vi "CAN.Cleanup.vi"(8 "error in (no error)":errorcluster, 11 "State Variables Out":T1 {"ADCS Connection"."RX_DL" items=["8"=8, "12"=12, "16"=16, "20"=20, "24"=24, "32"=32, "48"=48, "64"=64]; "ADCS Connection"."TX_DL" items=["8"=8, "12"=12, "16"=16, "20"=20, "24"=24, "32"=32, "48"=48, "64"=64]; "ADCS Connection"."I/O Mode" items=["CAN", "CAN FD", "CAN FD+BRS"]; "Parameters"."Properties"."Writes"."Signals"."Byte Order" items=["Little Endian", "Big Endian"]; "Parameters"."Properties"."Writes"."Signals"."Data Type" items=["Signed", "Unsigned", "IEEE Float"]; "Parameters"."Properties"."CAN"."IO Mode" items=["CAN 2.0", "CAN FD", "CAN FD+BRS"]; "Parameters"."Properties"."CAN"."Fill Byte" format="%.0x"; "Parameters"."Properties"."CAN"."VW TP Channel ID" format="%.0x"; "Parameters"."Properties"."CAN"."Receive UUDT ID" format="%.0x"; "Parameters"."Properties"."CAN"."Receive Extension" format="%.0x"; "Parameters"."Properties"."CAN"."Transmit Extension" format="%.0x"; "Parameters"."Properties"."CAN"."Receive ID" format="%.0x"; "Parameters"."Properties"."CAN"."Transmit ID" format="%.0x"; "Parameters"."Properties"."Reads"."Signals"."Byte Order" items=["Little Endian", "Big Endian"]; "Parameters"."Properties"."Reads"."Signals"."Data Type" items=["Signed", "Unsigned", "IEEE Float"]}) -> (0 "error out":errorcluster)   [LabVIEW 2015, in "Diagnostics Addon Engine.lvlib"]
uses:
  Diagnostics Addon Engine.lvlib
  Types/Diagnostics.State.ctl
  <vilib>/NI/NIVS Addon Network Comm/Engine/VeriStand Comm.lvclass
  <vilib>/NI/NIVS Inline Async API/_VS Inline Async API/Process/Process.lvclass
  Shared/Types/SysDef.Compile.ctl
  Shared/Types/SysDef.Compile.Properties.ctl
  Shared/Types/CAN.ctl
  Shared/Types/CAN.Interface.ctl
  Shared/Types/Protocol.ctl
  Shared/Types/Transport.ctl
  Shared/Types/Security.ctl
  Shared/Types/986x.ctl
  Shared/Types/Frame.Compile.ctl
  Shared/Types/Type.ctl
  Shared/Types/Signal.ctl
  Shared/Types/DPID.ctl
  Shared/Types/DPID.Rate.ctl
  Shared/Types/DTC.Settings.ctl
  Shared/Types/DTC.Descriptor.ctl
  <vilib>/Automotive Diagnostic Command Set/Diagnostic Transport.llb/Diag Reference.ctl
  <vilib>/Automotive Diagnostic Command Set/Diagnostic Transport.llb/Transport Protocol Selector.ctl
  Types/XNET.Refs.ctl
  <vilib>/NI/AMC/Message Queue.ctl
  <vilib>/NI/AMC/Message.ctl
  <vilib>/NI/Tools/Keyed Array/KeyedArray.ctl
  <vilib>/NI/NIVS Inline Async API/_Data Access Engine/Data Access Engine/Types/Write.DVR.ctl
  <vilib>/NI/NIVS Inline Async API/_Data Access Engine/Access Type Classes/Write/Write.lvclass
  <vilib>/NI/NIVS Inline Async API/_Data Access Engine/Data Access Engine/Types/Read.DVR.ctl
  <vilib>/NI/NIVS Inline Async API/_Data Access Engine/Access Type Classes/Read/Read.lvclass
  <vilib>/NI/NIVS Inline Async API/_Data Access Engine/Data Access Engine/Types/ReadWrite.DVR.ctl
  <vilib>/NI/NIVS Inline Async API/_Data Access Engine/Access Type Classes/ReadWrite/ReadWrite.lvclass
  <vilib>/NI/NIVS Inline Async API/_Data Access Engine/Access Type Classes/Write/Write.lvclass/Write.ctl
  <vilib>/NI/NIVS Inline Async API/_Data Access Engine/Data Access Engine/Methods/Write.Data.vi
  <vilib>/NI/NIVS Inline Async API/_Data Access Engine/Access Type Classes/Write/Write.ProcessData.vi
  ADCS.Get.ErrorByte.vi
  <vilib>/xnet/xnet.llb/XNET Database Close (Database).vi
  <vilib>/xnet/xnet.llb/XNET Database Delete (Cluster).vi
  Shared/SubVIs/Constants.vi
  <vilib>/addons/Automotive Diagnostic Command Set/NI_Automotive Diagnostic Command Set.lvlib
  <vilib>/NI VeriStand/Custom Device Tools/Custom Device Utility Library/Custom Device Utility Library.lvlib
  <vilib>/NI/NIVS Inline Async API/_Data Access Engine/Data Access Engine/Data Access Engine.lvclass
  Shared/Diagnostics Addon Shared.lvlib
  <vilib>/NI/Tools/Keyed Array/Tools_KeyedArray.lvlib
  <vilib>/NI/AMC/AMC.lvlib
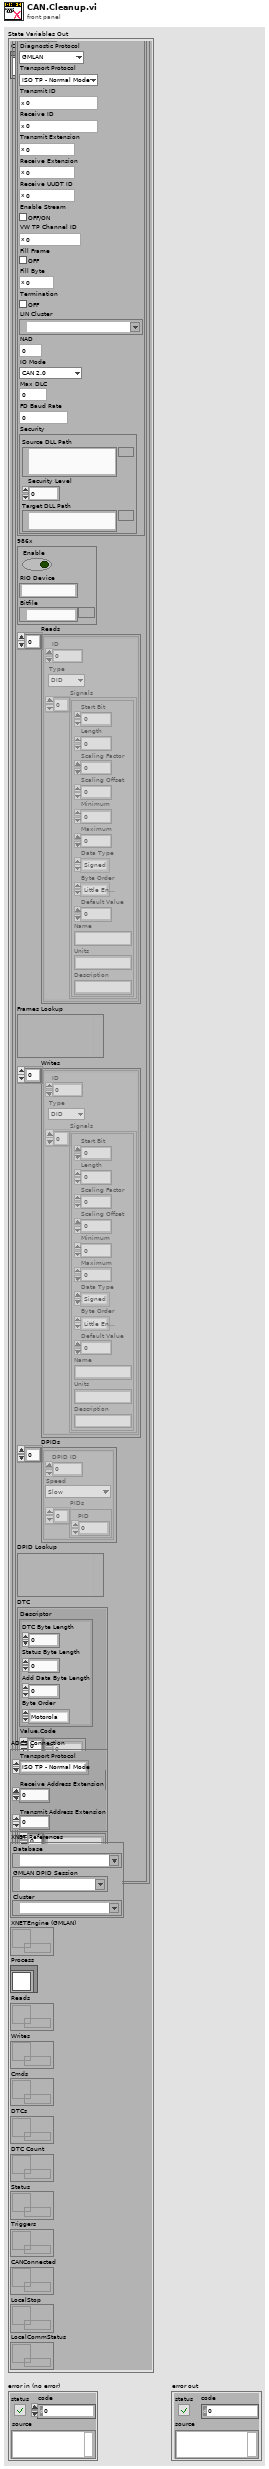
[diagram p1: front panel]
types:
  T1 = typedef "Diagnostics Addon Engine.lvlib/Diagnostics.State.ctl" = cluster{"Comm":refnum<class "VeriStand Comm.lvclass">, "Parameters":T2, "ADCS Connection":T17, "XNET References":T19, "XNETEngine (GMLAN)":T20, "Process":refnum<class "Process.lvclass">, "Reads":T21, "Writes":T22, "Cmds":T23, "DTCs":T21, "DTC Count":T21, "Status":T21, "Triggers":T23, "CANConnected":T21, "LocalStop":refnum<data-value>, "LocalCommStatus":refnum<data-value>}
  T2 = typedef "Diagnostics Addon Shared.lvlib/SysDef.Compile.ctl" = cluster{"Properties":T3}
  T3 = typedef "Diagnostics Addon Shared.lvlib/SysDef.Compile.Properties.ctl" = cluster{"Name":string, "CAN":T4, "986x":T9, "Reads":T10[], "Frames Lookup":variant, "Writes":T10[], "DPIDs":T13[], "DPID Lookup":variant, "DTC":T15, "Created DTCs":u32}
  T4 = typedef "Diagnostics Addon Shared.lvlib/CAN.ctl" = cluster{"Interface":T5, "Baud Rate":u32, "Diagnostic Protocol":T6, "Transport Protocol":T7, "Transmit ID":u32, "Receive ID":u32, "Transmit Extension":u8, "Receive Extension":u8, "Receive UUDT ID":u32, "Enable Stream":bool, "VW TP Channel ID":u32, "Fill Frame":bool, "Fill Byte":u8, "Termination":bool, "LIN Cluster":refnum<k21>, "NAD":u8, "IO Mode":u32, "Max DLC":u16, "FD Baud Rate":u32, "Security":T8}
  T5 = typedef "Diagnostics Addon Shared.lvlib/CAN.Interface.ctl" = string
  T6 = typedef "Diagnostics Addon Shared.lvlib/Protocol.ctl" = enum16{"GMLAN", "KWP-2000", "UDS", "User-Defined"}
  T7 = typedef "Diagnostics Addon Shared.lvlib/Transport.ctl" = enum16{"ISO TP - Normal Mode", "ISO TP - Mixed Mode", "VW TP 2.0", "Diagnostics on IP", "ISO TP LIN"}
  T8 = typedef "Diagnostics Addon Shared.lvlib/Security.ctl" = cluster{"Source DLL Path":path, "Security Level":u8, "Target DLL Path":path}
  T9 = typedef "Diagnostics Addon Shared.lvlib/986x.ctl" = cluster{"Enable":bool, "RIO Device":string, "Bitfile":path}
  T10 = typedef "Diagnostics Addon Shared.lvlib/Frame.Compile.ctl" = cluster{"ID":u32, "Type":T11, "Signals":T12[]}
  T11 = typedef "Diagnostics Addon Shared.lvlib/Type.ctl" = enum16{"DID", "CDID", "PID", "CPID", "Read Memory", "Write Memory", "DTC Control", "IO Cmd", "IO Resp", "Routine Start Cmd", "Routine Start Resp", "Routine Request Cmd", "Routine Request Resp", "Routine Stop Cmd", "Routine Stop Resp", "UserDefined Cmd", "UserDefined Rsp"}
  T12 = typedef "Diagnostics Addon Shared.lvlib/Signal.ctl" = cluster{"Start Bit":u32, "Length":u32, "Scaling Factor":dbl, "Scaling Offset":dbl, "Minimum":dbl, "Maximum":dbl, "Data Type":u32, "Byte Order":u32, "Default Value":dbl, "Name":string, "Units":string, "Description":string}
  T13 = typedef "Diagnostics Addon Shared.lvlib/DPID.ctl" = cluster{"DPID ID":u8, "Speed":T14, "PIDs":u16[]}
  T14 = typedef "Diagnostics Addon Shared.lvlib/DPID.Rate.ctl" = enum16{"Slow", "Medium", "Fast"}
  T15 = typedef "Diagnostics Addon Shared.lvlib/DTC.Settings.ctl" = cluster{"Descriptor":T16, "Value.Code":dbl[], "Value.String":string[], "Status.Code":dbl[], "Status.String":string[]}
  T16 = typedef "Diagnostics Addon Shared.lvlib/DTC.Descriptor.ctl" = cluster{"DTC Byte Length":i32, "Status Byte Length":i32, "Add Data Byte Length":i32, "Byte Order":enum16{"Motorola", "Intel"}}
  T17 = typedef "NI_Automotive Diagnostic Command Set.lvlib/Diag Reference.ctl" = cluster{"Diag CAN Handle":u32, "Transport Protocol":T18, "Receive Address Extension":u8, "Transmit Address Extension":u8, "Receive CAN Id":u32, "Transmit CAN Id":u32, "Log Frames ?":bool, "My TP Address":u8, "Other TP Address":u8, "T1":u16, "T2":u16, "T3":u16, "T4":u16, "Tx SN":u8, "Block Size":u8, "Rx SN":u8, "VW TP Initialized?":bool, "Tx block no":u8, "baud rate":u64, "Interface":string, "Channel Diag CAN Handle":u32, "UDP Connection ID":refnum<k16>, "TCP Connection ID":refnum<k5>, "Target IP Addr":u32, "Source Address":u16, "Target Address":u16, "Send Header NACK?":bool, "DLL Handle":u32, "NAD":u8, "Time Stamp read first":dbl, "Time Stamp read last":dbl, "Time Stamp write first":dbl, "Time Stamp write last":dbl, "Time Stamp write":dbl, "Time Stamp read":dbl, " I/O Mode":u32, "FD Baudrate":u64, "TX_DL":u16, "RX_DL":u16}
  T18 = typedef "NI_Automotive Diagnostic Command Set.lvlib/Transport Protocol Selector.ctl" = enum16{"ISO TP - Normal Mode", "ISO TP - Mixed Mode", "VW TP 2.0", "Diagnostics on IP", "ISO TP LIN"}
  T19 = typedef "Diagnostics Addon Engine.lvlib/XNET.Refs.ctl" = cluster{"Database":refnum<k21>, "GMLAN DPID Session":refnum<k21>, "Cluster":refnum<k21>}
  T20 = typedef "AMC.lvlib/Message Queue.ctl" = refnum<queue>
  T21 = typedef "Data Access Engine.lvlib/Data Access Engine.lvclass/Write.DVR.ctl" = refnum<data-value>
  T22 = typedef "Data Access Engine.lvlib/Data Access Engine.lvclass/Read.DVR.ctl" = refnum<data-value>
  T23 = typedef "Data Access Engine.lvlib/Data Access Engine.lvclass/ReadWrite.DVR.ctl" = refnum<data-value>
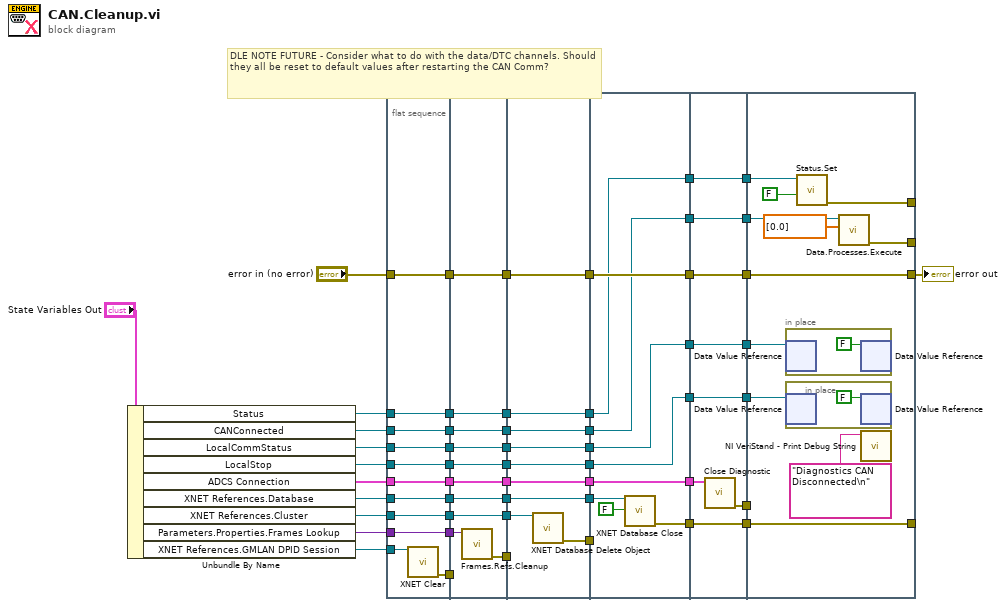
[diagram p0: block diagram]
diagram:
  # "DLE NOTE FUTURE - Consider what to do with the data/DTC channels. Should they all be reset to default values after restarting the CAN Comm?"
  n1 = Unbundle By Name("State Variables Out") -> ("Status"=w11:T21, "CANConnected"=w10:T21, "LocalCommStatus"=w12:refnum<data-value>, "LocalStop"=w9:refnum<data-value>, "ADCS Connection"=w5:T17, "XNET References.Database"=w4:refnum<k21>, "XNET References.Cluster"=w3:refnum<k21>, "Parameters.Properties.Frames Lookup"=w2:variant, "XNET References.GMLAN DPID Session"=w1:refnum<k21>)
  n2 = flat-sequence {
    tunnel: w3 -> [w63]
    tunnel: w2 -> [w64]
    tunnel: [w64] -> w53
    tunnel: [w63] -> w52
    tunnel: w1 -> [w62]
    tunnel: [w61] -> w51
    tunnel: [w60] -> w50
    tunnel: w5 -> [w60]
    tunnel: [w59] -> w49
    tunnel: w4 -> [w59]
    tunnel: "error in (no error)" -> [w58]
    tunnel: [w58] -> w48
    tunnel: [w57] -> w47
    tunnel: w9 -> [w57]
    tunnel: [w56] -> w46
    tunnel: w10 -> [w56]
    tunnel: [w55] -> w45
    tunnel: w11 -> [w55]
    tunnel: w12 -> [w54]
    tunnel: [w54] -> w44
    tunnel: [w74] -> w43
    tunnel: w53 -> [w73]
    tunnel: w52 -> [w74]
    tunnel: w51 -> [_]
    tunnel: [w72] -> w42
    tunnel: w50 -> [w72]
    tunnel: [w71] -> w41
    tunnel: w49 -> [w71]
    tunnel: [w70] -> w40
    tunnel: [w69] -> w39
    tunnel: w48 -> [w69]
    tunnel: [w68] -> w38
    tunnel: w47 -> [w68]
    tunnel: [w67] -> w37
    tunnel: w46 -> [w67]
    tunnel: [w66] -> w36
    tunnel: w45 -> [w66]
    tunnel: [w65] -> w35
    tunnel: w44 -> [w65]
    tunnel: w43 -> [w82]
    tunnel: [w83] -> w34
    tunnel: w42 -> [w83]
    tunnel: [w81] -> w33
    tunnel: w41 -> [w81]
    tunnel: [w80] -> w32
    tunnel: w40 -> [_]
    tunnel: [w79] -> w31
    tunnel: w39 -> [w79]
    tunnel: [w78] -> w30
    tunnel: w38 -> [w78]
    tunnel: [w77] -> w29
    tunnel: w37 -> [w77]
    tunnel: [w76] -> w28
    tunnel: w36 -> [w76]
    tunnel: [w75] -> w27
    tunnel: w35 -> [w75]
    tunnel: [w90] -> w26
    tunnel: w34 -> [w92]
    tunnel: [w92] -> w25
    tunnel: w33 -> [w91]
    tunnel: w32 -> [_]
    tunnel: [w88] -> w24
    tunnel: w31 -> [w88]
    tunnel: [w87] -> w23
    tunnel: w30 -> [w87]
    tunnel: [w86] -> w22
    tunnel: w29 -> [w86]
    tunnel: [w85] -> w21
    tunnel: w28 -> [w85]
    tunnel: [w84] -> w20
    tunnel: w27 -> [w84]
    tunnel: w26 -> [w100]
    tunnel: w25 -> [w99]
    tunnel: w24 -> [w98]
    tunnel: [w100] -> w19
    tunnel: [w98] -> w18
    tunnel: [w97] -> w17
    tunnel: [w96] -> w16
    tunnel: w23 -> [w96]
    tunnel: w22 -> [w95]
    tunnel: [w95] -> w15
    tunnel: [w94] -> w14
    tunnel: w21 -> [w94]
    tunnel: [w93] -> w13
    tunnel: w20 -> [w93]
    tunnel: [w110] -> w8
    tunnel: [w111] -> _
    tunnel: w19 -> [w111]
    tunnel: w18 -> [w110]
    tunnel: w17 -> [_]
    tunnel: w16 -> [w108]
    tunnel: w15 -> [w106]
    tunnel: w14 -> [w105]
    tunnel: [w103] -> _
    tunnel: [w102] -> _
    tunnel: w13 -> [w101]
    frame #0 {
      n3 = call <vilib>:"XNET Clear.vi"("session in"=w62) -> ("error out"=w61:errorcluster)  [unwired: 14 in]
    }
    frame #1 {
      n4 = call "Frames.Refs.Cleanup.vi"("Lookup"=w73) -> ("Array"=w70:errorcluster[])  [unwired: 10 in]
    }
    frame #2 {
      n5 = call-poly <vilib>:"XNET Database Delete Object.vi"("cluster in"=w82) -> ("error out"=w80:errorcluster)  [unwired: 14 in]
    }
    frame #3 {
      n6 = call-poly <vilib>:"XNET Database Close.vi"("database in"=w91, "close all? (true)"=FALSE) -> ("error out"=w90:errorcluster)  [unwired: 13 in]
    }
    frame #4 {
      n7 = call <vilib>:"Close Diagnostic.vi"("diag ref in"=w99) -> ("error out"=w97:errorcluster)  [unwired: 10 in]
    }
    frame #5 {
      n8 = in-place {
        n9 = in-place-dvr #1(w101) -> ()  [unwired: 2 out]
        n10 = in-place-dvr #1(FALSE ("data value")) -> ()  [unwired: 2 out]
      }
      n11 = in-place {
        n12 = in-place-dvr #2(w108) -> ()  [unwired: 2 out]
        n13 = in-place-dvr #2(FALSE ("data value")) -> ()  [unwired: 2 out]
      }
      n14 = call "Status.Set.vi"("success?"=FALSE ("Boolean"), "Status Ref"=w105) -> ("error out"=w103:errorcluster)  [unwired: 9 in]
      n15 = call-poly <vilib>:"Data.Processes.Execute.vi"("Values"=dbl[] [0.0], "Ref"=w106) -> ("error out"=w102:errorcluster)  [unwired: 9 in]
      n16 = call <vilib>:"NI VeriStand - Print Debug String.vi"("Message"="Diagnostics CAN Disconnected\n") -> ()  [unwired: 10 in, 1 out]
    }
  }
  "error out" <- w8
